vi "Mark Initialized.vi"(8 "error in (no error)":errorcluster, 11 "device in":refnum<class "NI_Robotics_Starter Kit Base Device.lvclass">) -> (0 "error out":errorcluster, 3 "device out":refnum<class "NI_Robotics_Starter Kit Base Device.lvclass">)   [LabVIEW 2017, in "NI_Robotics_Starter Kit Base Device.lvclass"]
uses:
  <vilib>/robotics/Starter Kit/Base Device/NI_Robotics_Starter Kit Base Device.lvclass
  <vilib>/robotics/Starter Kit/Base Device/NI_Robotics_Starter Kit Base Device.lvclass/NI_Robotics_Starter Kit Base Device.ctl
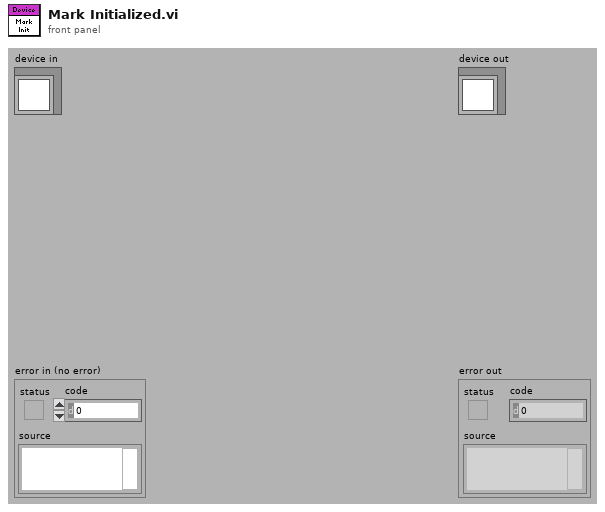
[diagram p1: front panel]
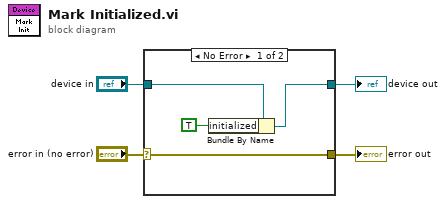
[diagram p0: block diagram]
diagram:
  n1 = case shown="No Error" "error in (no error)" {
    selector: "error in (no error)" -> [w8 w10]
    tunnel: [w8 w10] -> w3
    tunnel: [w6 w9] -> w1
    tunnel: "device in" -> [w7 w9]
    frame No Error {
      n2 = Bundle By Name(cluster=w7, "initialized"=TRUE) -> (w6:refnum<class "NI_Robotics_Starter Kit Base Device.lvclass">)
    }
    frame Error {
    }
  }
  "error out" <- w3
  "device out" <- w1
